vi "ConvertValiseData.vi"(4 "entrée d'erreur":errorcluster caption="entrée d'erreur (pas d'erreur)", 7 "NomProjet":string) -> (0 "sortie d'erreur":errorcluster, 3 "ProjetOUT":string)   [LabVIEW 2017]
uses:
  DefDeType/WhichPath.ctl
panel:
  out "size(s)":i32
  out "Waveform Graph":waveform(dbl)[](graph)
  out "taille(s)":i32[](array[numeric])
  out "Tableau":dbl[][](array[numeric])
  out "floor(x/y)":i32
  out "taille(s) 2":i32
  out "données":waveform(dbl)[](array[waveform])
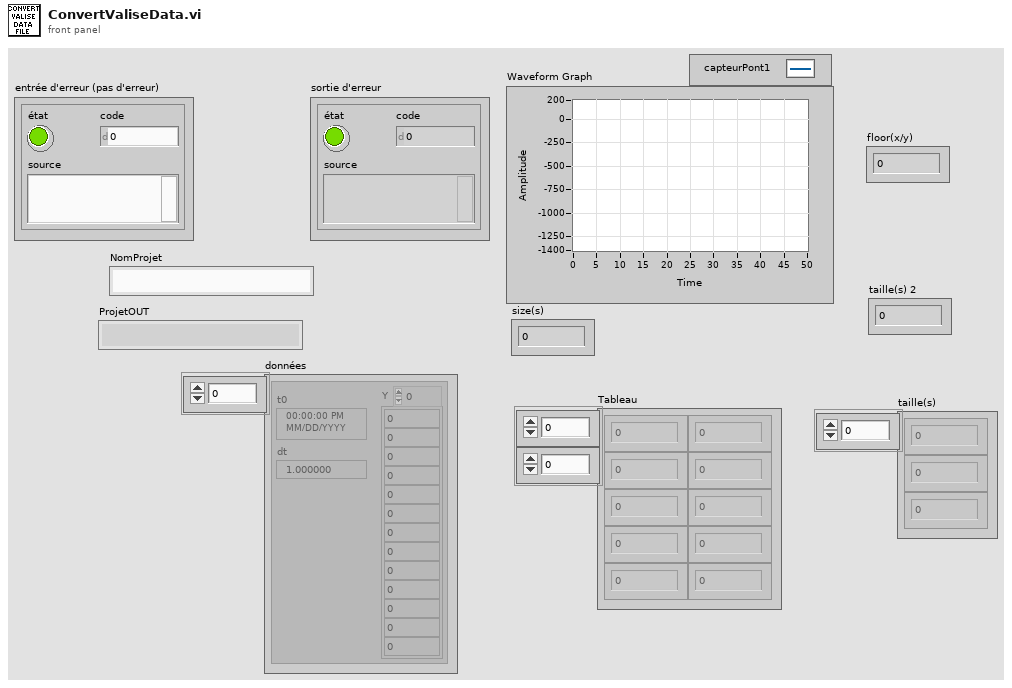
[diagram p1: front panel]
types:
  T1 = typedef "WhichPath.ctl" = enum16{"DossierProjet", "Config", "Meas", "MeasSuitCase", "MeasOnBoard", "MeasQualisys", "MeasTDMS", "MeasHexapode", "MeasNortek", "Fig", "Res", "MeasUSB"}
  T2 = enum16{"open", "open or create", "create or replace", "create", "open (read-only)"}
  T3 = typedef "ConfigTotale.ctl" = cluster{"VoltageChannels":T4, "WheastoneBridgeChannels":T5, "Configuration":T6}
  T4 = typedef "VoltageChannels.ctl" = cluster{"ChannelNames":string[], "Sensitivity(Unit/V)":dbl[], "AutoZero":bool[], "ChannelUnits":string[], "Offsets(Units)":dbl[], "Graph Num":u8[]}
  T5 = typedef "WBridgeChannels.ctl" = cluster{"ChannelNames":string[], "Sensitivity(Unit/V)":dbl[], "AutoZero":bool[], "ChannelUnits":string[], "Offsets(Units)":dbl[], "Graph Num":u8[]}
  T6 = typedef "Configuration.ctl" = cluster{"AcqSamplingRate(Hz)":u32, "AcqTime(s)":u32, "Trigger":bool, "NbVoltageChannels":u32, "NbWBridgeChannels":u32, "Qualisys":bool, "Hexapode":bool, "FinalSamplingRate(Hz)":u32, "QualisysDataType":enum16{"6DOF", "3DTracking", "6DOF + 3D"}, "Nortek":bool}
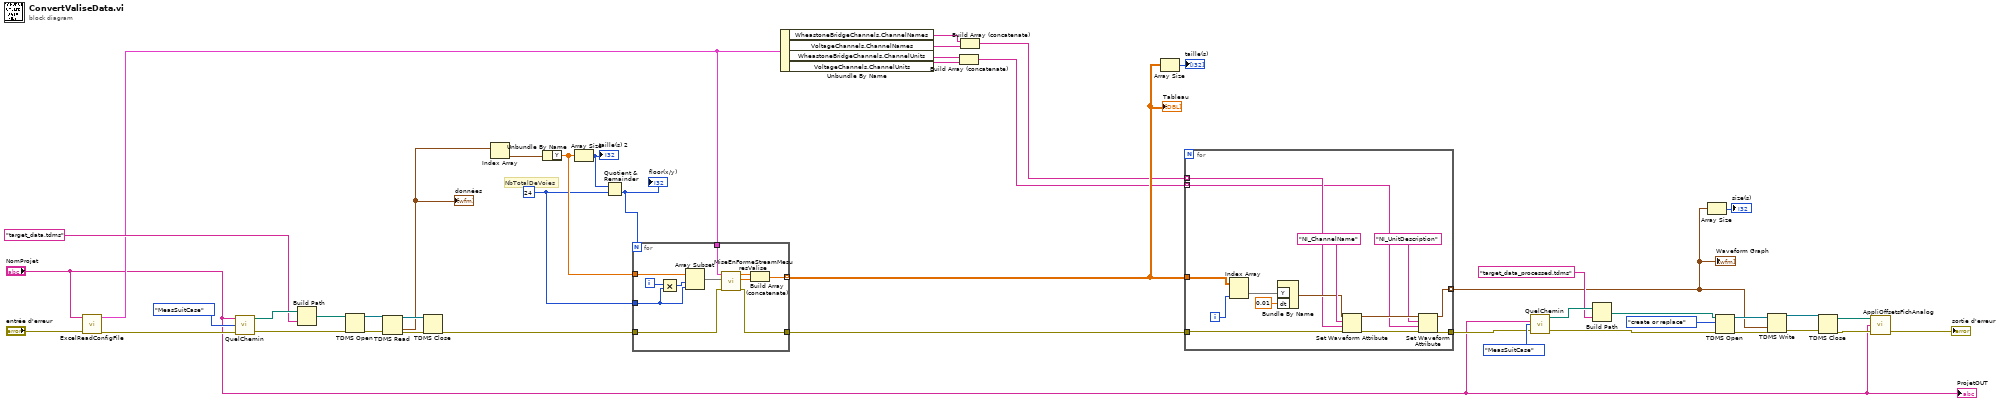
[diagram p0: block diagram]
diagram:
  w11 = 24 ("y")
  # "NbTotalDeVoies"
  n1 = call "ExcelReadConfigFile.vi"("NomProjet"="NomProjet", "error in (no error)"="entrée d'erreur") -> ("ConfigurationTotale"=w10:T3, "error out"=w13:errorcluster)  [unwired: 3 in]
  n2 = call "QuelChemin.vi"("Entrée d'erreur"=w13, "WhichPath?"=WhichPath."MeasSuitCase", "NomProjet"="NomProjet") -> ("Sortie d'erreur"=w25:errorcluster, "SurDisqueLocal"=w27:path)  [unwired: 1 out]
  n3 = Build Path(base path=w27, name or relative path="target_data.tdms" ("username")) -> (appended path=w24:path)
  n4 = TDMS Open(8:w25, 11:w24) -> (0:w44:errorcluster, 3:w45:refnum<k34>)  [unwired: 5 in]
  n5 = TDMS Read(0:w45, 11:w44) -> (4:w43:refnum<k34>, 10:w12:waveform(dbl)[], 15:w42:errorcluster)  [unwired: 6 in, 3 out]
  "données" <- w12
  n6 = TDMS Close(8:w42, 11:w43) -> (0:w35:errorcluster)  [unwired: 1 out]
  n7 = Index Array(array=w12) -> (element=w41:waveform(dbl))  [unwired: 1 in]
  n8 = Unbundle By Name(w41) -> ("Y"=w38:dbl[])
  n9 = Array Size(array=w38) -> (size(s)=w40:i32)
  "taille(s) 2" <- w40
  n10 = Quotient & Remainder(x=w40, y=w11) -> (floor(x/y)=w39:i32)  [unwired: 1 out]
  "floor(x/y)" <- w39
  n11 = for {
    N: w39 -> [_]
    tunnel: w38 -> [w56]
    tunnel: [w48] -> w36 mode=indexing
    tunnel: w35 -> [w52]
    tunnel: [w51] -> w34
    tunnel: w11 -> [w53]
    tunnel: w10 -> [w49]
    i -> [w55]
    n12 = Multiply(x=w55, y=w53) -> (x*y=w54:i32)
    n13 = Array Subset(array=w56, index=w54, length=w53) -> (w50:dbl[])
    n14 = call "MiseEnFormeStreamMesuresValise.vi"("Error In"=w52, "MesuresBrutesValise"=w50, "ConfigTotale"=w49) -> ("Error Out"=w51:errorcluster, "VoltageChannels1(0to15)"=w46:dbl[], "WBridgeChannels"=w47:dbl[])  [unwired: 2 in]
    n15 = Build Array (concatenate)(w47, w46) -> (w48:dbl[])
  }
  "Tableau" <- w36
  n16 = Unbundle By Name(w10) -> ("WheastoneBridgeChannels.ChannelNames"=w9:string[], "VoltageChannels.ChannelNames"=w8:string[], "WheastoneBridgeChannels.ChannelUnits"=w7:string[], "VoltageChannels.ChannelUnits"=w6:string[])
  n17 = Build Array (concatenate)(w7, w6) -> (w4:string[])
  n18 = Build Array (concatenate)(w9, w8) -> (w5:string[])
  n19 = Array Size(array=w36) -> (size(s)=→"taille(s)":i32[])
  n20 = for {
    tunnel: w36 -> [w70]
    tunnel: [w59] -> w2 mode=indexing
    tunnel: w34 -> [w62]
    tunnel: [w61] -> w20
    tunnel: w5 -> [w58] mode=indexing
    tunnel: w4 -> [w57] mode=indexing
    i -> [w69]
    n21 = Index Array(array=w70, index (col)=w69) -> (element=w68:dbl[])  [unwired: 1 in]
    n22 = Bundle By Name("Y"=w68, "dt"=0.01) -> (w60:waveform(dbl))  [unwired: 1 in]
    n23 = Set Waveform Attribute(4:w62, 5:w58, 6:"NI_ChannelName" ("nom"), 7:w60) -> (0:w65:errorcluster, 3:w66:waveform(dbl))  [unwired: 1 out]
    n24 = Set Waveform Attribute(4:w65, 5:w57, 6:"NI_UnitDescription" ("nom"), 7:w66) -> (0:w61:errorcluster, 3:w59:waveform(dbl))  [unwired: 1 out]
  }
  "Waveform Graph" <- w2
  n25 = call "QuelChemin.vi"("Entrée d'erreur"=w20, "WhichPath?"=WhichPath."MeasSuitCase", "NomProjet"="NomProjet") -> ("Sortie d'erreur"=w19:errorcluster, "SurDisqueLocal"=w22:path)  [unwired: 1 out]
  n26 = Build Path(base path=w22, name or relative path="target_data_processed.tdms" ("username")) -> (appended path=w18:path)
  n27 = Array Size(array=w2) -> (size(s)=→"size(s)":i32)
  n28 = TDMS Open(8:w19, 10:T2."create or replace" ("opération (0 : open)"), 11:w18) -> (0:w32:errorcluster, 3:w31:refnum<k34>)  [unwired: 4 in]
  n29 = TDMS Write(0:w31, 9:w2, 11:w32) -> (4:w29:refnum<k34>, 15:w30:errorcluster)  [unwired: 3 in, 2 out]
  n30 = TDMS Close(8:w30, 11:w29) -> (0:w17:errorcluster, 3:w15:path)
  n31 = call "AppliOffsetsFichAnalog.vi"("entrée d'erreur"=w17, "NomProjet"="NomProjet", "CheminFichier"=w15) -> ("sortie d'erreur"=→"sortie d'erreur":errorcluster)  [unwired: 1 in, 1 out]
  "ProjetOUT" <- "NomProjet"
